vi "Get Tamer Logo.vi"() -> (0 "Tamer Logo":picture)   [LabVIEW 2020, in "Tamer.lvlib" / "Tamer.lvclass"]
uses:
  Tamer.lvclass
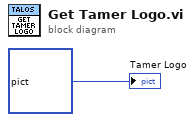
[diagram p0: block diagram]
diagram:
  "Tamer Logo" <- picture bytes[12830] ("Tamer Picture 2")
